vi "Next PV Data.vi"(8 "error in (no error)":errorcluster, 9 "timeout":dbl[unit]=1.0, 11 "Subscription in":refnum<class "Subscription.lvclass">) -> (0 "error out":errorcluster, 1 "timed out?":bool, 2 "PV Data":refnum<class "PV Data.lvclass">, 3 "Subscription out":refnum<class "Subscription.lvclass">, 5 "PV name":string)   [LabVIEW 2020, in "PV Access.lvlib" / "PVA Client.lvlib" / "Subscription.lvclass"]
uses:
  Subscription.lvclass
  PV Data/PV Data/PV Data.lvclass
  PV Access.lvlib
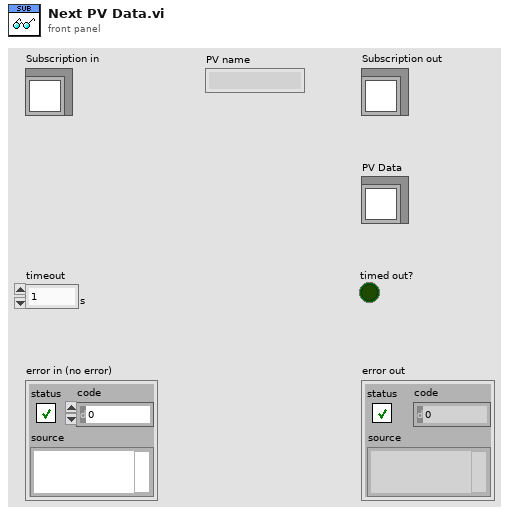
[diagram p1: front panel]
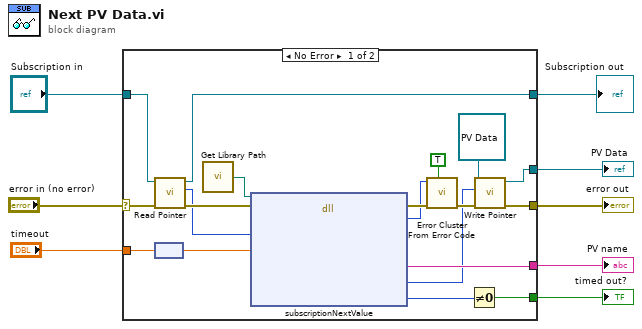
[diagram p0: block diagram]
diagram:
  n1 = case shown="No Error" "error in (no error)" {
    selector: "error in (no error)" -> [w26 w28]
    tunnel: [w10 w28] -> w7
    tunnel: [w23 w29] -> w5
    tunnel: "Subscription in" -> [w24 w29]
    tunnel: "timeout" -> [w18 _]
    tunnel: [w9 _] -> w4
    tunnel: [w20 _] -> w3
    tunnel: [w14 _] -> w1
    frame No Error {
      n2 = call-dynamic "Read Pointer.vi"("error in (no error)"=w26, "Pointer Base in"=w24) -> ("error out"=w25:errorcluster, "Pointer"=w22:i64, "Pointer Base out"=w23:refnum<class "Subscription.lvclass">)  [unwired: 7 in]
      n3 = node(w18) -> (w19:dbl)
      n4 = call "Get Library Path.vi"() -> ("Path"=w27:path)  [unwired: 1 in]
      n5 = dll-call lib="?" fn="subscriptionNextValue"(path in=w27, error in=w25, "subscription"=w22, "timeout"=w19) -> (error out=w16:errorcluster, "ret_code"=w15:i32, "pvName"=w14:string, "value"=w11:i64, "timedOut"=w21:i16)  [unwired: 6 in, 1 out]
      n6 = call <vilib>:"Error Cluster From Error Code.vi"("show call chain? (False)"=TRUE, "error in (no error)"=w16, "error code (0)"=w15) -> ("error out"=w13:errorcluster)  [unwired: 6 in]
      n7 = Not Equal To 0?(x=w21) -> (x != 0?=w20:bool)
      n8 = call-dynamic "Write Pointer.vi"("error in (no error)"=w13, "Pointer"=w11, "Pointer Base in"=refnum<class "PV Data.lvclass"> refnum ("PV Access.lvlib:PV Data.lvlib:PV Data.lvclass")) -> ("error out"=w10:errorcluster, "Pointer Base out"=w9:refnum<class "PV Data.lvclass">)  [unwired: 7 in]
    }
    frame Error {
    }
  }
  "error out" <- w7
  "Subscription out" <- w5
  "timed out?" <- w3
  "PV Data" <- w4
  "PV name" <- w1
